vi "LinTFine_Scan.vi"() -> ()   [LabVIEW 2019]
uses:
  Light Field/lightfield-automation-labview/LightField Automation.lvclass
panel:
  out "Spectrum":cluster{"Array 2":dbl[], "Array":dbl[]}(graph)
  out "LightField Automation error out":errorcluster
  out "LightField Automation out":refnum<class "LightField Automation.lvclass">
  out "number":i32
  out "output string":string
  in  "PZC200 Instrument Channel":string="GPIB/0:4,0"
  in  "Acq Time (ms)":dbl=500.0 caption="Acq Time :" min=0.0 max=360000.0 step=50.0
  in  "LinTFines Step Pos (usteps)":dbl=1.0 caption="Step pos (usteps)" min=1.0 max=100.0 step=1.0
  in  "LinTFine End Pos (usteps)":dbl=10.0 caption="End pos (usteps)" min=-1000000.0 max=1000000.0 step=1.0
  in  "LinTFine Start Pos (usteps)":dbl caption="Start pos (usteps)" min=-1000000.0 max=1000000.0 step=1.0
  # "ms"
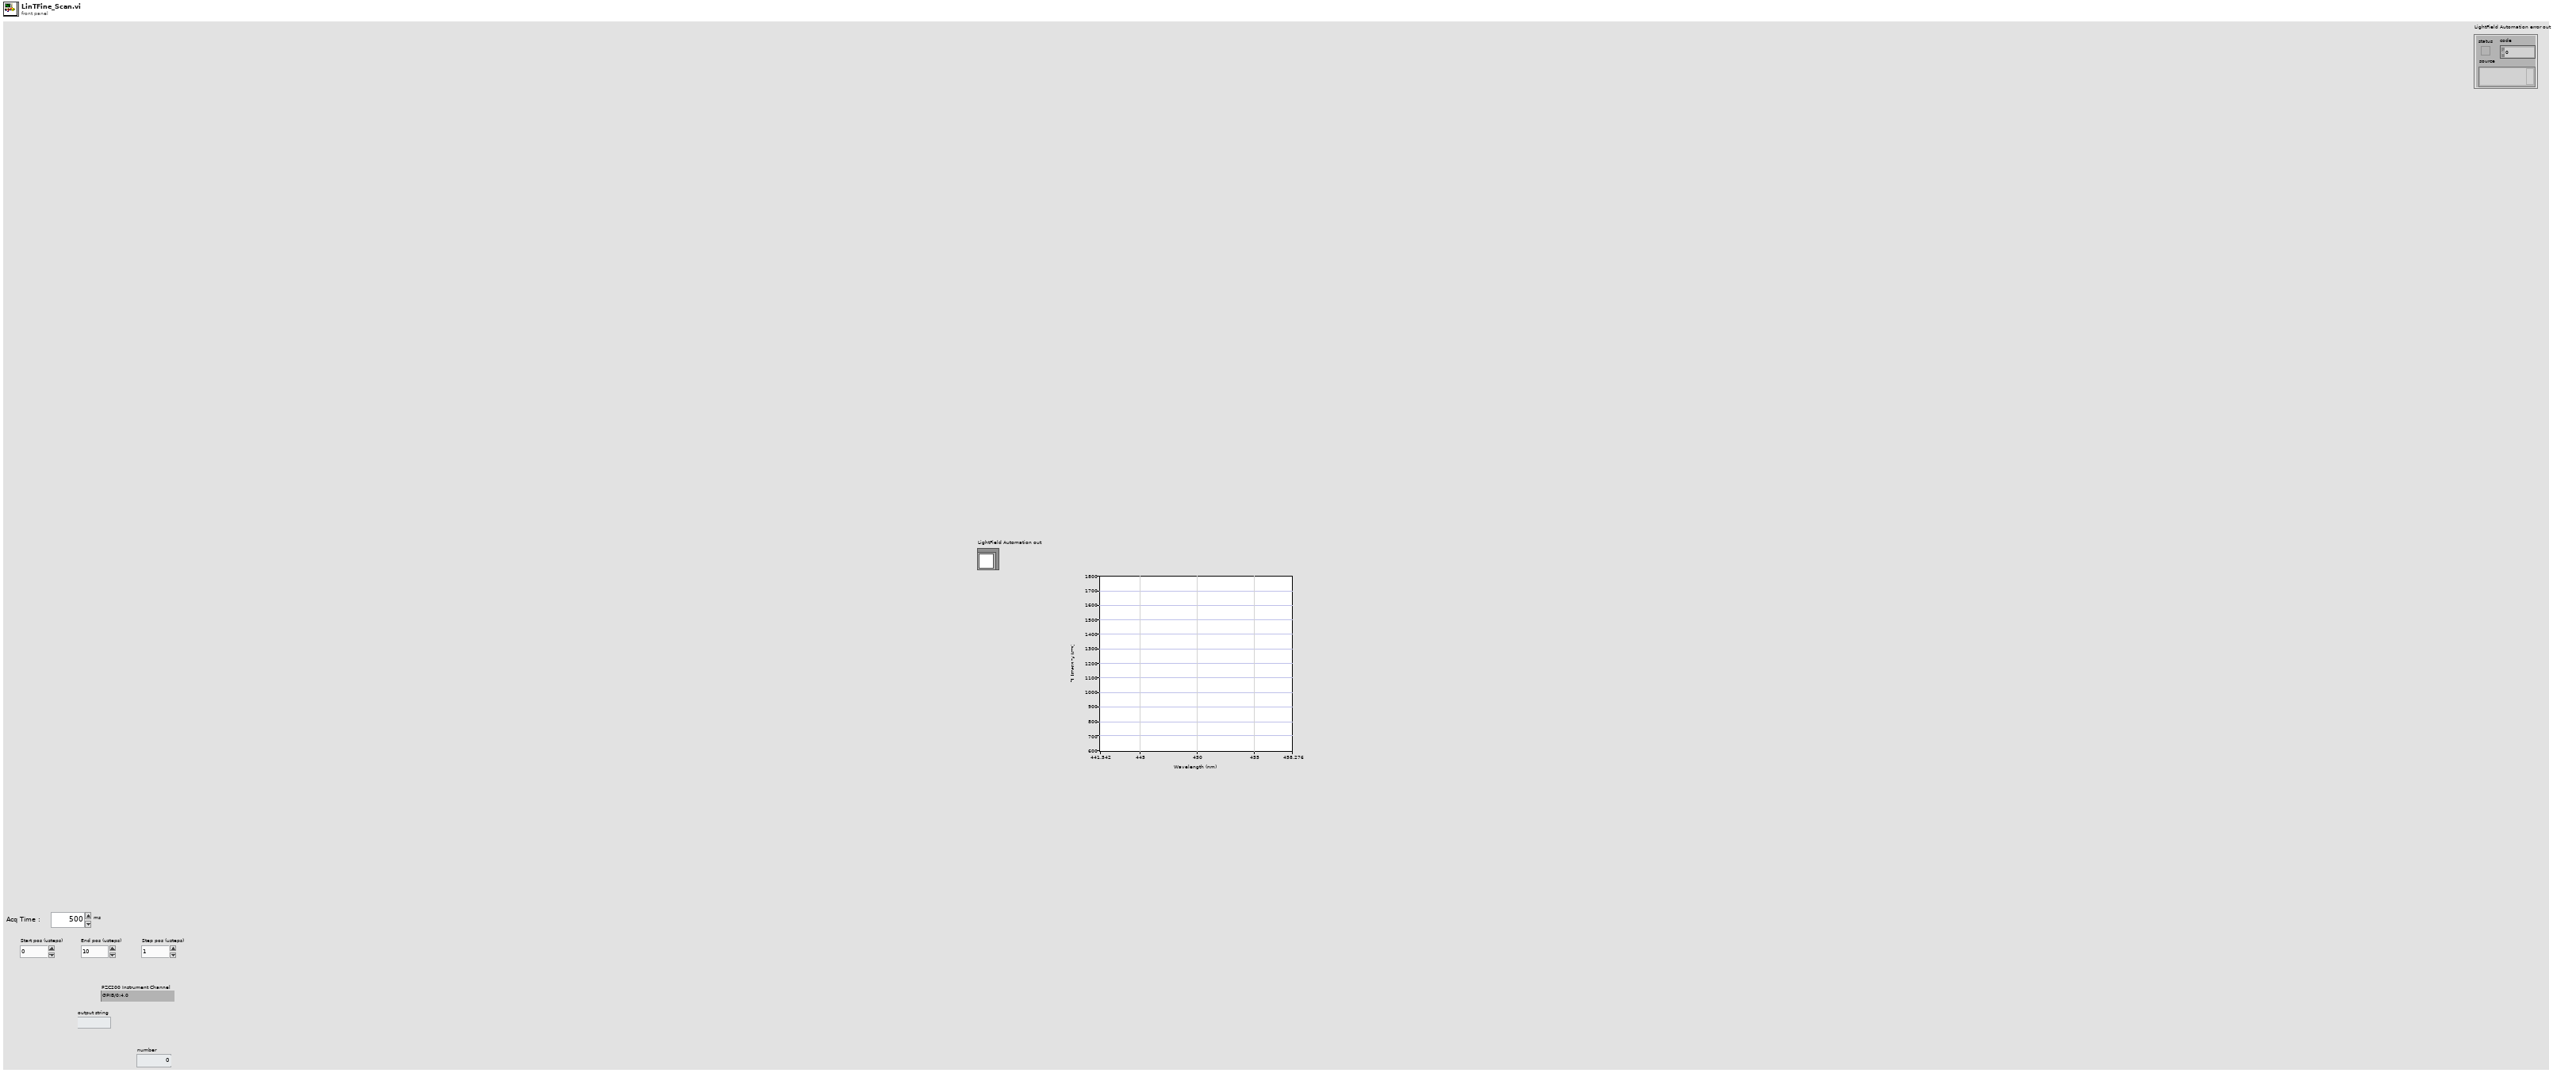
[diagram p1: front panel]
types:
  T1 = enum16{"Image", "Spectrum", "APD 1", "APD 2", "APD 1+2"}
  T2 = enum16{"Spectre", "Polarisation", "XY Intensity Map"}
  T3 = cluster{"Image":dbl[][][], "Frame Size":cluster{"F":i32, "Y":i32, "X":i32}}[]
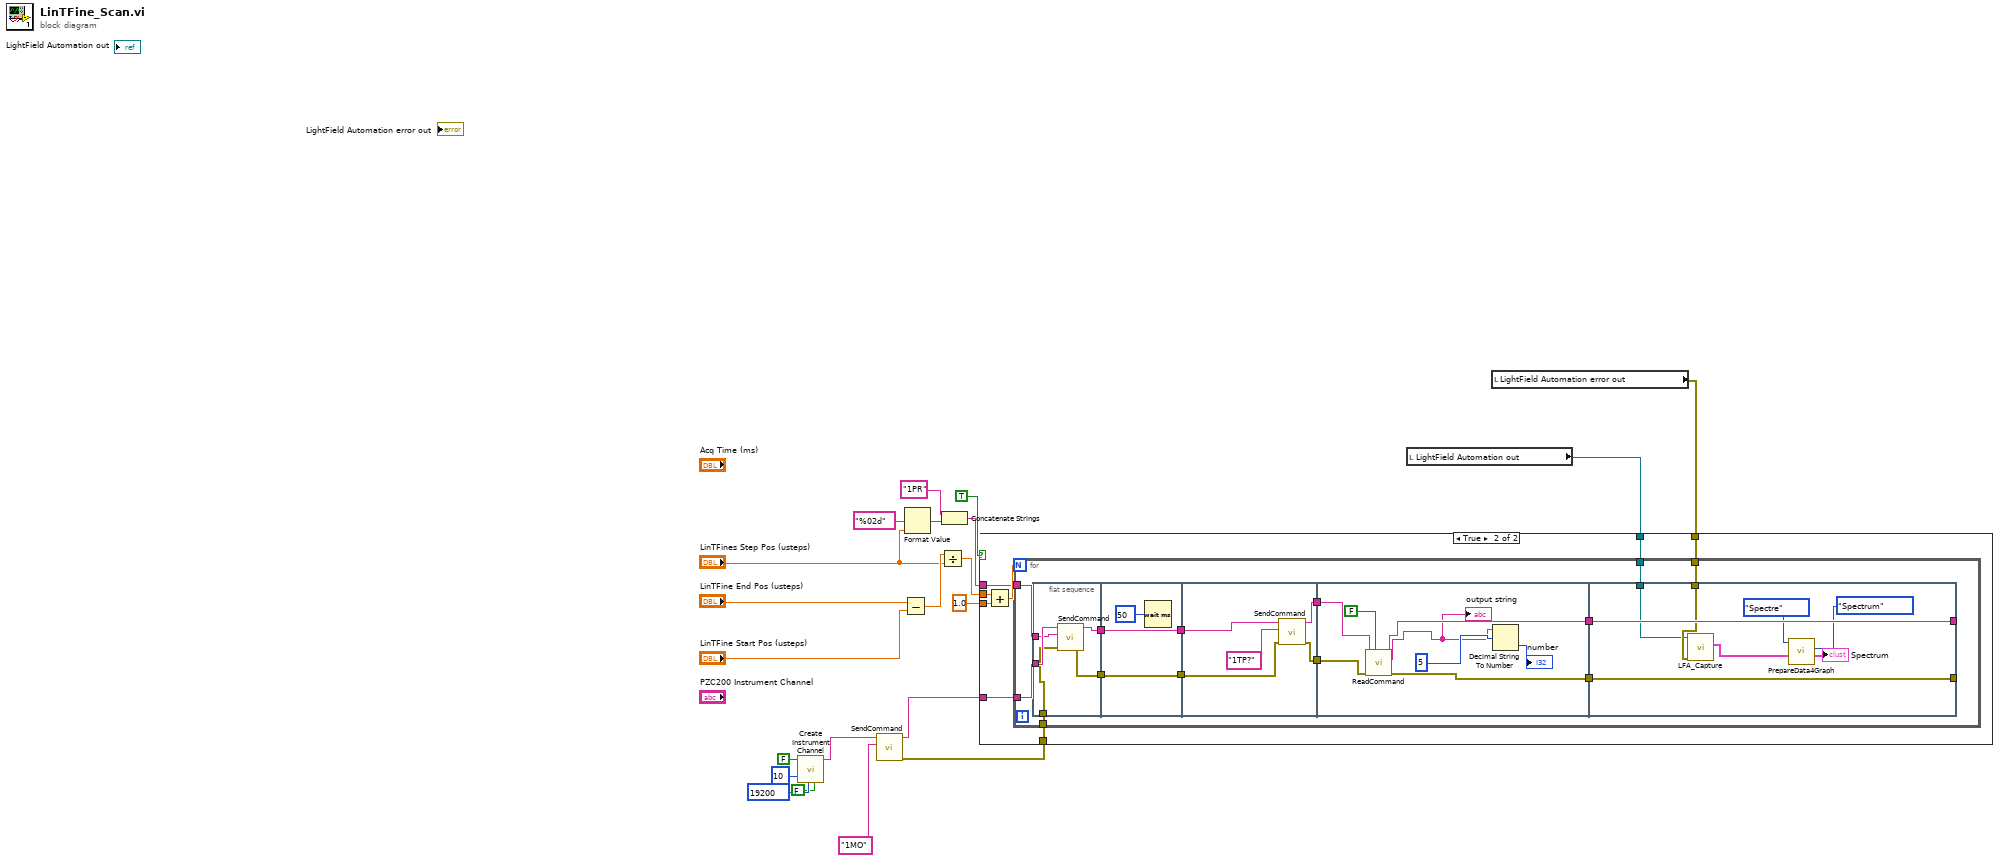
[diagram p0: block diagram]
diagram:
  n1 = call "Create Instrument Channel.vi"("XON/XOFF Handshaking(F)"=FALSE, "Baud Rate (38400)"=u32 19200, "COM Port (1)"=u8 10, "(T) - GPIB, F - RS232"=FALSE) -> ("Instrument Channel out"=w6:string)  [unwired: 5 in, 2 out]
  n2 = call "SendCommand.vi"("Command"="1MO", "Instrument Channel"=w6) -> ("error out"=w4:errorcluster, "Instrument Channel out"=w5:string)  [unwired: 8 in]
  n3 = Subtract(x="LinTFine End Pos (usteps)", y="LinTFine Start Pos (usteps)") -> (x-y=w19:dbl)
  n4 = Format Value(format string="%02d", value (0)="LinTFines Step Pos (usteps)") -> (output string=w12:string)  [unwired: 1 in]
  n5 = Divide(x=w19, y="LinTFines Step Pos (usteps)") -> (x/y=w18:dbl)
  n6 = Concatenate Strings("1PR", w12) -> (w11:string)
  n7 = local read "LightField Automation out"() -> (w1:refnum<class "LightField Automation.lvclass">)
  n8 = local read "LightField Automation error out"() -> (w2:errorcluster)
  n9 = case shown="True" TRUE {
    tunnel: w18 -> [_ w29]
    tunnel: 1.0 ("y") -> [_ w28]
    tunnel: w5 -> [_ w25]
    tunnel: w11 -> [_ w26]
    tunnel: w4 -> [_ w24]
    tunnel: w2 -> [_ w23]
    tunnel: w1 -> [_ w22]
    frame False {
    }
    frame True {
      n10 = Add(x=w29, y=w28) -> (x+y=w27:dbl)
      n11 = for {
        N: w27 -> [_]
        tunnel: w25 -> [w42]
        tunnel: w26 -> [w41]
        tunnel: w24 -> [w32]
        tunnel: w23 -> [w31]
        tunnel: w22 -> [w30]
        n12 = flat-sequence {
          tunnel: w42 -> [w47]
          tunnel: w41 -> [w46]
          tunnel: [w45] -> w40
          tunnel: [w44] -> w37
          tunnel: w32 -> [w43]
          tunnel: w40 -> [w49]
          tunnel: [w49] -> w39
          tunnel: [w48] -> w38
          tunnel: w37 -> [w48]
          tunnel: w39 -> [w55]
          tunnel: w38 -> [w54]
          tunnel: [w52] -> w36
          tunnel: [w51] -> w35
          tunnel: w36 -> [w63]
          tunnel: w35 -> [w62]
          tunnel: [w59] -> w34
          tunnel: [w60] -> w33
          tunnel: [w70] -> _
          tunnel: [w71] -> _
          tunnel: w34 -> [w71]
          tunnel: w33 -> [w70]
          tunnel: w31 -> [w69]
          tunnel: w30 -> [w68]
          frame #0 {
            n13 = call "SendCommand.vi"("error in"=w43, "Command"=w46, "Instrument Channel"=w47) -> ("error out"=w44:errorcluster, "Instrument Channel out"=w45:string)  [unwired: 7 in]
          }
          frame #1 {
            n14 = Wait (ms)(milliseconds to wait=u32 50) -> ()  [unwired: 1 out]
          }
          frame #2 {
            n15 = call "SendCommand.vi"("error in"=w54, "Command"="1TP?", "Instrument Channel"=w55) -> ("error out"=w52:errorcluster, "Instrument Channel out"=w51:string)  [unwired: 7 in]
          }
          frame #3 {
            n16 = call "ReadCommand.vi"("Disable MAV check (F)"=FALSE, "error in"=w63, "Instrument Channel"=w62) -> ("error out"=w60:errorcluster, "Response"=w56:string, "Instrument Channel out"=w59:string)  [unwired: 6 in]
            "output string" <- w56
            n17 = Decimal String To Number(string=w56, offset=5 ("offset (0)")) -> (number=→"number":i32)  [unwired: 1 in, 1 out]
          }
          frame #4 {
            n18 = call "LFA_Capture.vi"("error in (no error)"=w69, "LightField Automation in"=w68) -> ("Data"=w65:T3)  [unwired: 7 in, 2 out]
            n19 = call "PrepareData4Graph.vi"("DataLF"=w65, "AcqMode"=T1."Spectrum", "Data type"=T2."Spectre") -> ("Spectrum"=→"Spectrum":cluster{"Array 2":dbl[], "Array":dbl[]})  [unwired: 5 in, 1 out]
          }
        }
      }
    }
  }
